vi "PerformMeasurement.vi"(8 "error in (no error)":errorcluster, 10 "gRPCid":T4, 11 "ctet_dmm":T1) -> (0 "error out":errorcluster, 3 "ctet_dmm out":T1)   [LabVIEW 2019, in "ctet_dmm User Library.lvlib"]
uses:
  ctet_dmm User Library.lvlib
  Servers/ctet_dmm/gRPC lvSupport/Server API/typeDefs/grpcId.ctl
  Types/ctet_dmm.ctl
  Servers/ctet_dmm/ctet_dmm Class/RPC Messages/measurementservice_DMMConfigResponse/measurementservice_DMMConfigResponse_Data.ctl
  Servers/ctet_dmm/ctet_dmm Class/RPC Messages/measurementservice_ErrorOut/measurementservice_ErrorOut_Data.ctl
  Servers/ctet_dmm/ctet_dmm Class/RPC Messages/measurementservice_DMMMeasurementData/measurementservice_DMMMeasurementData_Data.ctl
  Servers/ctet_dmm/ctet_dmm Class/ctet_dmm.lvclass
  Servers/ctet_dmm/gRPC lvSupport/gprc-lvsupport.lvlib
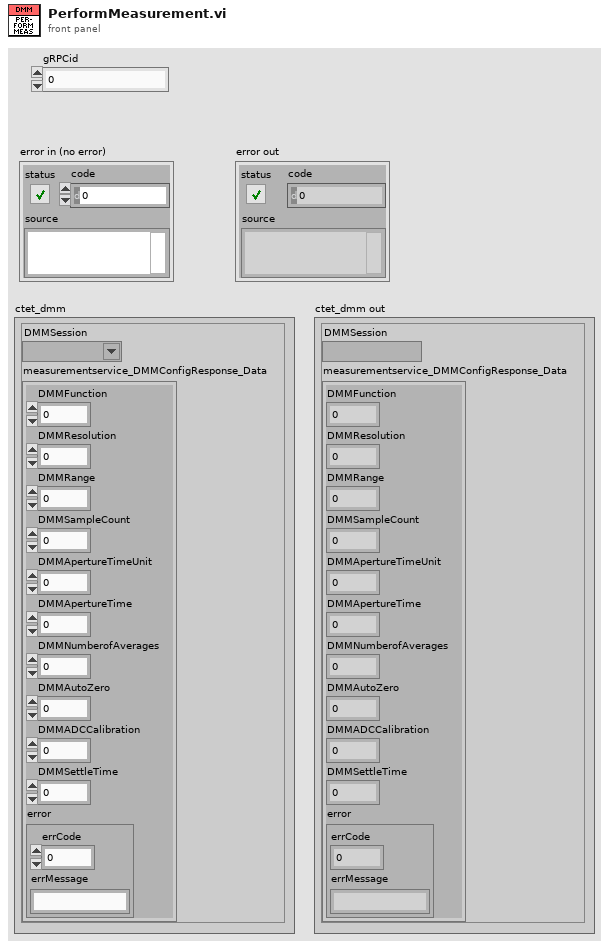
[diagram p1: front panel]
types:
  T1 = typedef "ctet_dmm User Library.lvlib/ctet_dmm.ctl" = cluster{"DMMSession":refnum<k15>, "measurementservice_DMMConfigResponse_Data":T2}
  T2 = typedef "ctet_dmm.lvlib/ctet_dmm.lvclass/measurementservice_DMMConfigResponse_Data.ctl" = cluster{"DMMFunction":i64, "DMMResolution":dbl, "DMMRange":dbl, "DMMSampleCount":i64, "DMMApertureTimeUnit":i64, "DMMApertureTime":dbl, "DMMNumberofAverages":i64, "DMMAutoZero":i64, "DMMADCCalibration":i64, "DMMSettleTime":dbl, "error":T3}
  T3 = typedef "ctet_dmm.lvlib/ctet_dmm.lvclass/measurementservice_ErrorOut_Data.ctl" = cluster{"errCode":i64, "errMessage":string}
  T4 = typedef "ctet_dmm.lvlib/gprc-lvsupport.lvlib/grpcId.ctl" = u64
  T5 = typedef "ctet_dmm.lvlib/ctet_dmm.lvclass/measurementservice_DMMMeasurementData_Data.ctl" = cluster{"measurement":dbl[], "error":T3}
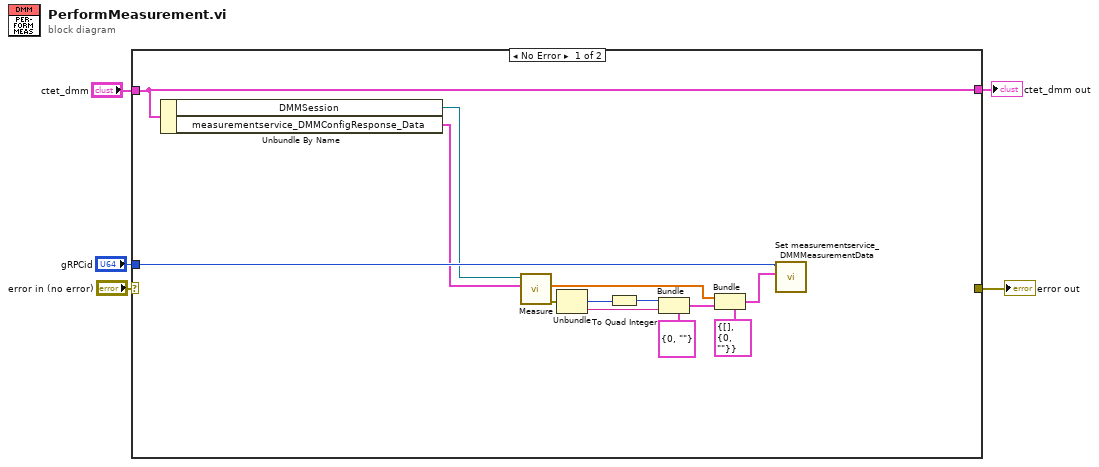
[diagram p0: block diagram]
diagram:
  n1 = case shown="No Error" "error in (no error)" {
    selector: "error in (no error)" -> [_ w20]
    tunnel: [_ w20] -> w5
    tunnel: "gRPCid" -> [w14 _]
    tunnel: "ctet_dmm" -> [w15 w19]
    tunnel: [w15 w19] -> w1
    frame No Error {
      n2 = Unbundle By Name(w15) -> ("DMMSession"=w9:refnum<k15>, "measurementservice_DMMConfigResponse_Data"=w7:T2)
      n3 = call "Measure.vi"("measurementservice_DMMConfigResponse_Data"=w7, "DMMSession"=w9) -> ("error out"=w8:errorcluster, "Measurements"=w6:dbl[])  [unwired: 8 in]
      n4 = Unbundle(w8) -> ("code"=w17:i32, "source"=w18:string)  [unwired: 1 out]
      n5 = To Quad Integer(1:w17) -> (0:w16:i64)
      n6 = Bundle(cluster=T3 {"errCode"=0, "errMessage"=""} ("error"), "errCode"=w16, "errMessage"=w18) -> (w12:T3)
      n7 = Bundle(cluster=T5 {"measurement"=[], "error"={"errCode"=0, "errMessage"=""}} ("measurementservice_DMMMeasurementData_Data"), "measurement"=w6, "error"=w12) -> (w10:T5)
      n8 = call "Set measurementservice_DMMMeasurementData.vi"("Message Data"=w10, "gRPCid"=w14) -> ()  [unwired: 9 in, 1 out]
    }
    frame Error {
    }
  }
  "error out" <- w5
  "ctet_dmm out" <- w1
